vi "Set_Gain_DDPCA-300.vi"(3 "error in":errorcluster, 4 "Status":i32, 5 "Gain [V/A]":T1(ring), 6 "index":i32) -> (0 "error out":errorcluster, 1 "Status_out":i32, 2 "index_out":i32)   [LabVIEW 2013, in "FEMTO_LUCI-10.lvlib"]
uses:
  FEMTO_LUCI-10.lvlib
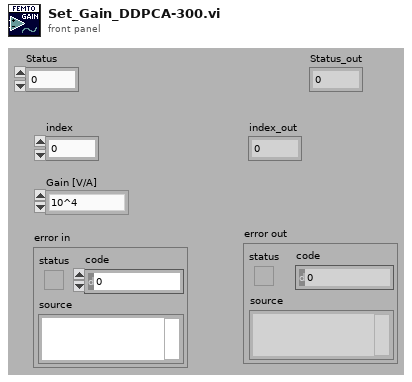
[diagram p1: front panel]
types:
  T1 = enum16{"10^4", "10^5", "10^6", "10^7", "10^8", "10^9", "10^10", "10^11", "10^12", "10^13"}
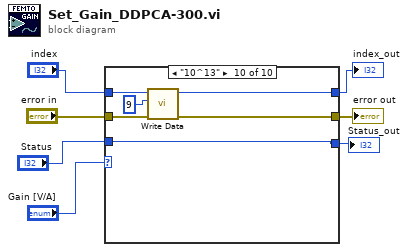
[diagram p0: block diagram]
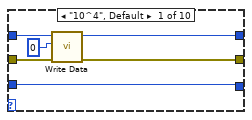
[diagram p2: hidden frame]
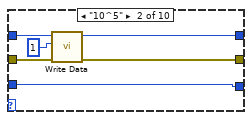
[diagram p3: hidden frame]
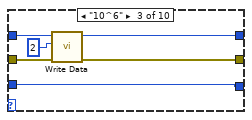
[diagram p4: hidden frame]
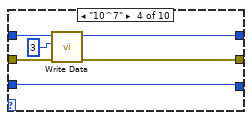
[diagram p5: hidden frame]
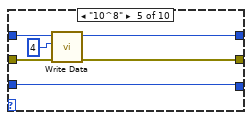
[diagram p6: hidden frame]
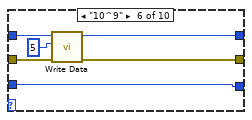
[diagram p7: hidden frame]
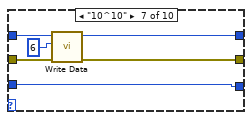
[diagram p8: hidden frame]
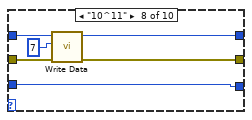
[diagram p9: hidden frame]
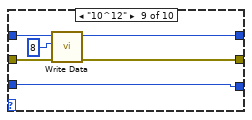
[diagram p10: hidden frame]
diagram:
  n1 = case shown="\"10^13\"" "Gain [V/A]" {
    tunnel: "index" -> [w10 w19 w22 w28 w34 w40 w46 w52 w59 w64]
    tunnel: "error in" -> [w13 w17 w25 w31 w37 w43 w49 w55 w61 w67]
    tunnel: [w12 w16 w24 w30 w36 w42 w48 w54 w60 w66] -> w6
    tunnel: [w9 w18 w23 w29 w35 w41 w47 w51 w58 w65] -> w7
    tunnel: "Status" -> [w8 w14 w20 w26 w32 w38 w44 w50 w56 w62]
    tunnel: [w8 w14 w20 w26 w32 w38 w44 w50 w56 w62] -> w1
    frame "10^4", Default {
      n2 = call "Write Data.vi"("error in (no error)"=w13, "data_low"=0, "index"=w10) -> ("error out"=w12:errorcluster, "index_out"=w9:i32)  [unwired: 1 in, 6 out]
    }
    frame "10^5" {
      n3 = call "Write Data.vi"("error in (no error)"=w17, "data_low"=1, "index"=w19) -> ("error out"=w16:errorcluster, "index_out"=w18:i32)  [unwired: 1 in, 6 out]
    }
    frame "10^6" {
      n4 = call "Write Data.vi"("error in (no error)"=w25, "data_low"=2, "index"=w22) -> ("error out"=w24:errorcluster, "index_out"=w23:i32)  [unwired: 1 in, 6 out]
    }
    frame "10^7" {
      n5 = call "Write Data.vi"("error in (no error)"=w31, "data_low"=3, "index"=w28) -> ("error out"=w30:errorcluster, "index_out"=w29:i32)  [unwired: 1 in, 6 out]
    }
    frame "10^8" {
      n6 = call "Write Data.vi"("error in (no error)"=w37, "data_low"=4, "index"=w34) -> ("error out"=w36:errorcluster, "index_out"=w35:i32)  [unwired: 1 in, 6 out]
    }
    frame "10^9" {
      n7 = call "Write Data.vi"("error in (no error)"=w43, "data_low"=5, "index"=w40) -> ("error out"=w42:errorcluster, "index_out"=w41:i32)  [unwired: 1 in, 6 out]
    }
    frame "10^10" {
      n8 = call "Write Data.vi"("error in (no error)"=w49, "data_low"=6, "index"=w46) -> ("error out"=w48:errorcluster, "index_out"=w47:i32)  [unwired: 1 in, 6 out]
    }
    frame "10^11" {
      n9 = call "Write Data.vi"("error in (no error)"=w55, "data_low"=7, "index"=w52) -> ("error out"=w54:errorcluster, "index_out"=w51:i32)  [unwired: 1 in, 6 out]
    }
    frame "10^12" {
      n10 = call "Write Data.vi"("error in (no error)"=w61, "data_low"=8, "index"=w59) -> ("error out"=w60:errorcluster, "index_out"=w58:i32)  [unwired: 1 in, 6 out]
    }
    frame "10^13" {
      n11 = call "Write Data.vi"("error in (no error)"=w67, "data_low"=9, "index"=w64) -> ("error out"=w66:errorcluster, "index_out"=w65:i32)  [unwired: 1 in, 6 out]
    }
  }
  "index_out" <- w7
  "error out" <- w6
  "Status_out" <- w1
